vi "Plot Observer.vi"(8 "error in (no error)":errorcluster, 11 "Vessel in":refnum<class "Vessel.lvclass">) -> (0 "error out":errorcluster, 3 "Vessel out":refnum<class "Vessel.lvclass">)   [LabVIEW 2014, in "Vessel.lvclass"]
doc: "This is the main running method that runs the control loop."
uses:
  Vessel.lvclass
panel:
  out "Gyro Bias":T1(graph)
  out "Yaw":cluster{"Numeric":dbl, "Numeric":dbl}(graph)
  out "Pitch":cluster{"Numeric":dbl, "Numeric":dbl}(graph)
  out "Roll":cluster{"Numeric":dbl, "Numeric":dbl}(graph)
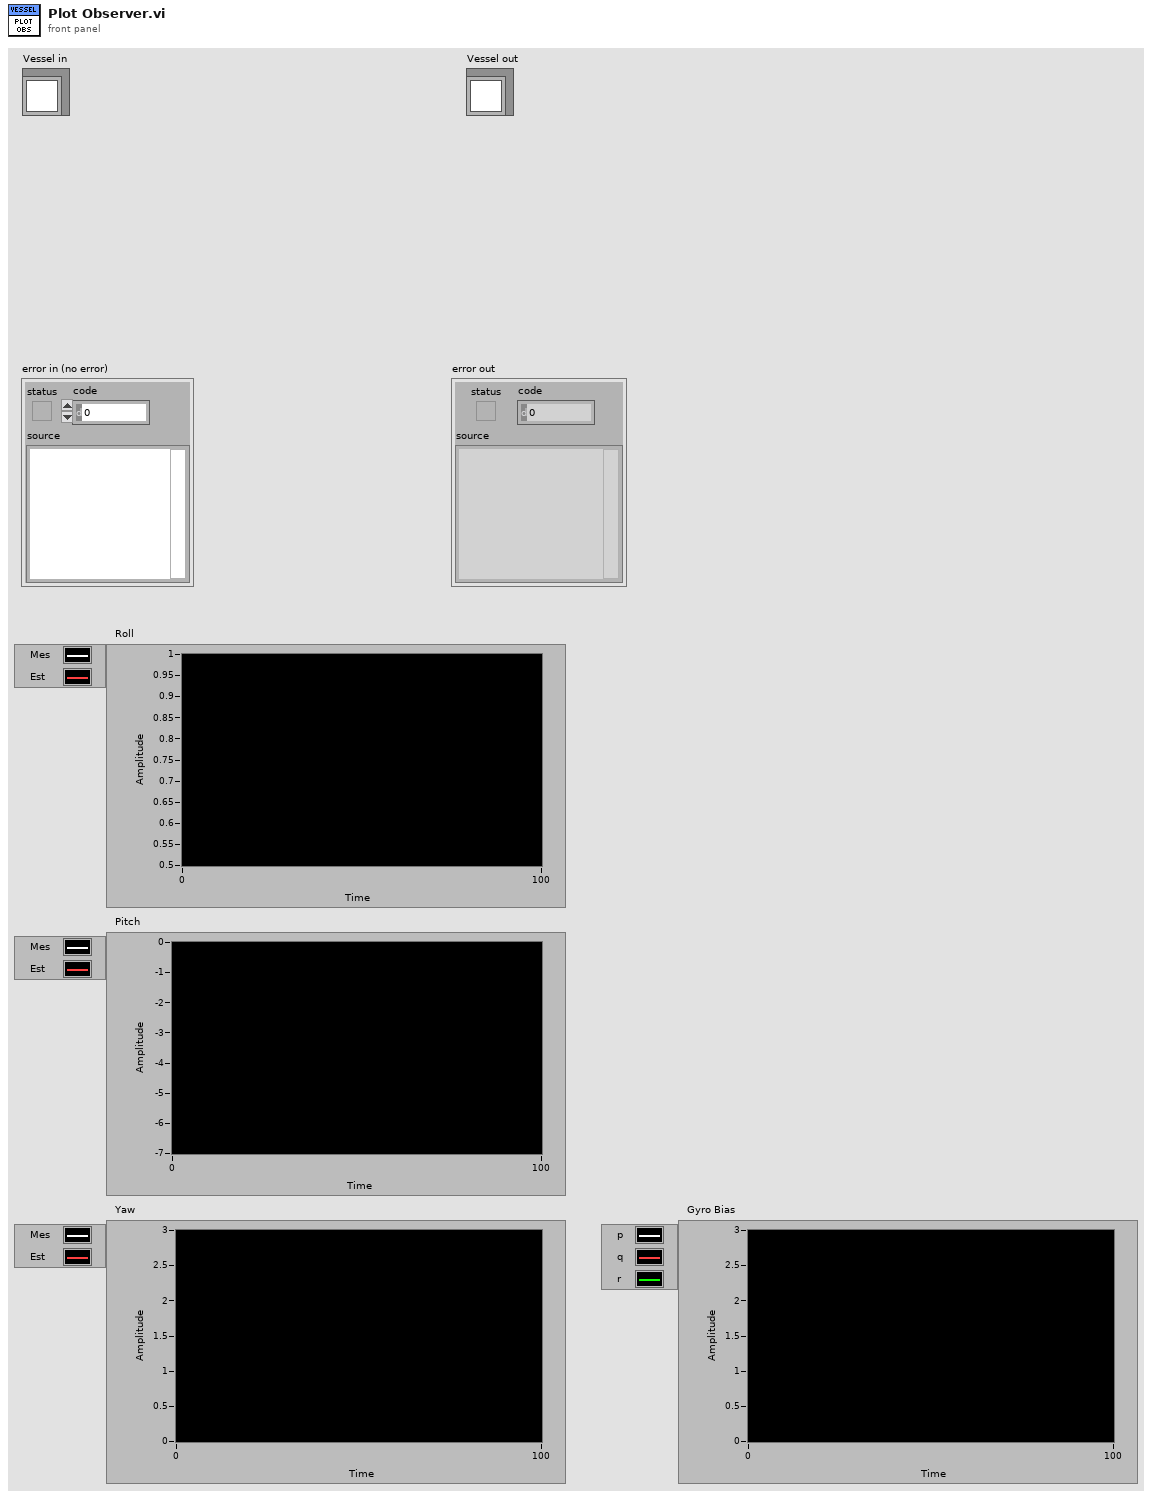
[diagram p1: front panel]
types:
  T1 = cluster{"Gyro Bias[0]":dbl, "Gyro Bias[1]":dbl, "Gyro Bias[2]":dbl, "Gyro Bias[3]":dbl, "Gyro Bias[4]":dbl, "Gyro Bias[5]":dbl, "Gyro Bias[6]":dbl, "Gyro Bias[7]":dbl, "Gyro Bias[8]":dbl}
  T2 = cluster{"Measured":cluster{"Eta":dbl[], "Nu":dbl[], "Eta Dot":dbl[], "Nu Dot":dbl[]}, "Estimated":cluster{"Eta":dbl[], "Nu":dbl[], "Eta Dot":dbl[], "Nu Dot":dbl[]}, "Desired":cluster{"Eta":dbl[], "Nu":dbl[], "Eta Dot":dbl[], "Nu Dot":dbl[]}, "Previous Desired":cluster{"Eta":dbl[], "Nu":dbl[], "Eta Dot":dbl[], "Nu Dot":dbl[]}, "tau":dbl[], "Altitude":cluster{"Measured":dbl, "Estimated":dbl, "Desired":dbl, "Previous Desired":dbl, "Approximated":dbl, "grad F":dbl[]}, "rpm":dbl[], "Attitude":cluster{"Theta Measured":dbl[], "Theta Estimated":dbl[], "Omega Measured":dbl[], "Omega Estimated":dbl[], "Gyro Bias":dbl[]}}
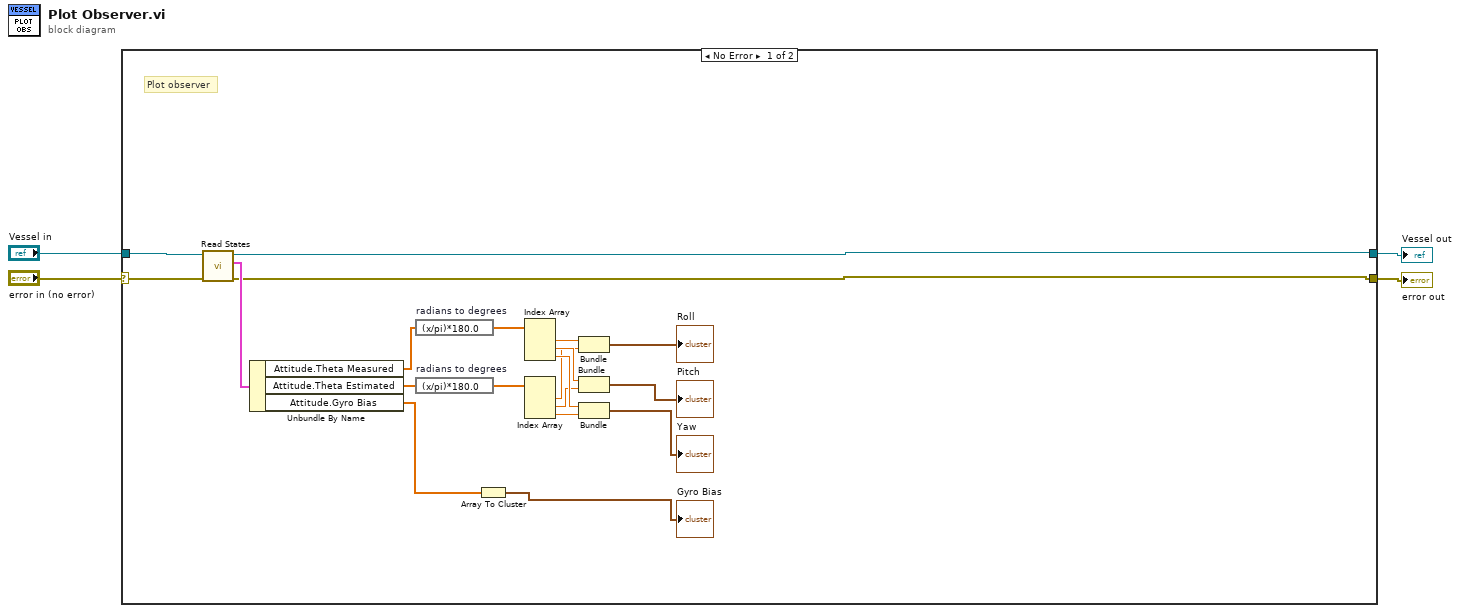
[diagram p0: block diagram]
diagram:
  n1 = case shown="No Error" "error in (no error)" {
    selector: "error in (no error)" -> [w23 w26]
    tunnel: [w20 w26] -> w3
    tunnel: [w21 w25] -> w1
    tunnel: "Vessel in" -> [w24 w25]
    frame No Error {
      # "Plot observer"
      n2 = call-dynamic "Read States.vi"("error in (no error)"=w23, "Vessel in"=w24) -> ("error out"=w20:errorcluster, "States"=w22:T2, "Vessel out"=w21:refnum<class "Vessel.lvclass">)  [unwired: 7 in]
      n3 = Unbundle By Name(w22) -> ("Attitude.Theta Measured"=w12:dbl[], "Attitude.Theta Estimated"=w10:dbl[], "Attitude.Gyro Bias"=w6:dbl[])
      n4 = expression code="(x/pi)*180.0" "radians to degrees"(w12) -> (w11:dbl[])
      n5 = expression code="(x/pi)*180.0" "radians to degrees"(w10) -> (w9:dbl[])
      n6 = Array To Cluster(array=w6) -> (cluster=→"Gyro Bias":T1)
      n7 = Index Array(array=w11) -> (element #1=w19:dbl, element #2=w18:dbl, element #3=w17:dbl)  [unwired: 3 in]
      n8 = Index Array(array=w9) -> (element #1=w16:dbl, element #2=w15:dbl, element #3=w14:dbl)  [unwired: 3 in]
      n9 = Bundle("Numeric"=w19, "Numeric"=w16) -> (→"Roll":cluster{"Numeric":dbl, "Numeric":dbl})  [unwired: 1 in]
      n10 = Bundle("Numeric"=w18, "Numeric"=w15) -> (→"Pitch":cluster{"Numeric":dbl, "Numeric":dbl})  [unwired: 1 in]
      n11 = Bundle("Numeric"=w17, "Numeric"=w14) -> (→"Yaw":cluster{"Numeric":dbl, "Numeric":dbl})  [unwired: 1 in]
    }
    frame Error {
    }
  }
  "error out" <- w3
  "Vessel out" <- w1
